vi "Check_config_file.vi"(8 "error in":errorcluster, 11 "path":path) -> (0 "error IO":errorcluster)   [LabVIEW 2019]
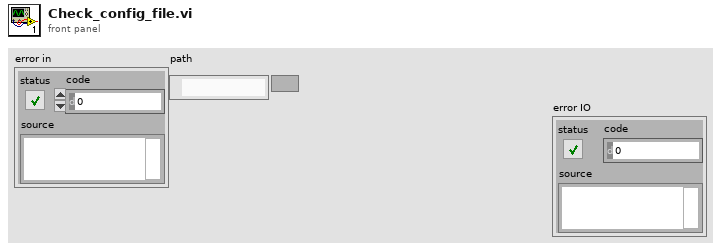
[diagram p1: front panel]
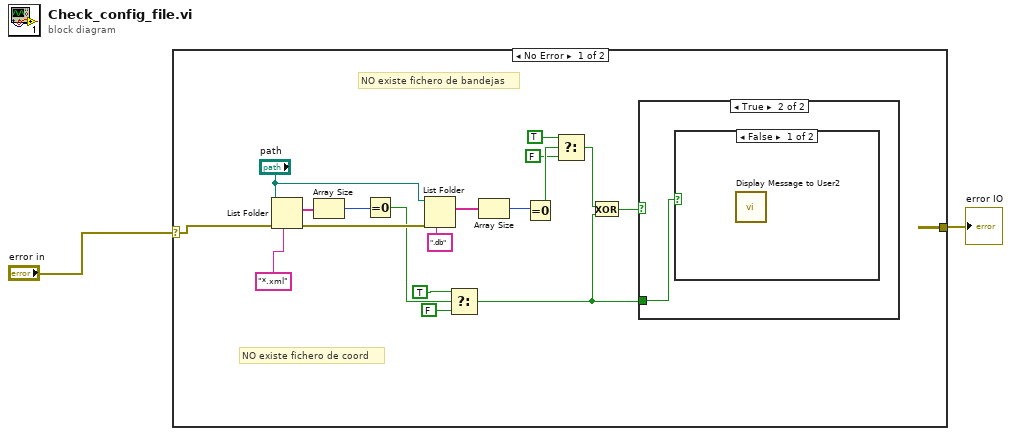
[diagram p0: block diagram]
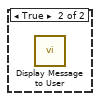
[diagram p3: hidden frame]
diagram:
  n1 = case shown="No Error" "error in" {
    selector: "error in" -> [w18 w22]
    tunnel: [_ w22] -> w1
    frame No Error {
      # "NO existe fichero de bandejas"
      # "NO existe fichero de coord"
      n2 = List Folder(path="path", pattern="*.xml", error in=w18) -> (filenames=w20:string[], error out=w16:errorcluster)  [unwired: 1 in, 2 out]
      n3 = Array Size(array=w20) -> (size(s)=w19:i32)
      n4 = Equal To 0?(x=w19) -> (x = 0?=w11:bool)
      n5 = List Folder(path="path", pattern=".db", error in=w16) -> (filenames=w14:string[])  [unwired: 1 in, 3 out]
      n6 = Select(t=TRUE, s=w11, f=FALSE) -> (s? t:f=w3:bool)
      n7 = Array Size(array=w14) -> (size(s)=w12:i32)
      n8 = Equal To 0?(x=w12) -> (x = 0?=w8:bool)
      n9 = Select(t=TRUE, s=w8, f=FALSE) -> (s? t:f=w4:bool)
      n10 = Exclusive Or(1:w3, 2:w4) -> (0:w5:bool)
      n11 = case shown="True" w5 {
        tunnel: w3 -> [_ w21]
        frame False {
        }
        frame True {
          n12 = case shown="False" w21 {
            frame False {
              n13 = call "Display Message to User2"() -> ()  [unwired: 10 in, 2 out]
            }
            frame True {
              n14 = call "Display Message to User"() -> ()  [unwired: 10 in, 2 out]
            }
          }
        }
      }
    }
    frame Error {
    }
  }
  "error IO" <- w1
